vi "SeCrTs-DO Start.vi"(8 "error in":errorcluster, 9 "DO config":T1(array[cluster]), 11 "Refnum in":refnum<k21>) -> (0 "error out":errorcluster, 3 "Refnum out":refnum<k21>)   [LabVIEW 2022 SP3]
doc: "This VI is for start for Analog Output"
uses:
  RT Controls/SeCrTs-FGV Read write.ctl
  <vilib>/DAQmx/configure/timing.llb/DAQmx Timing (Sample Clock).vi
  <vilib>/DAQmx/configure/trigger.llb/DAQmx Start Trigger (Digital Edge).vi
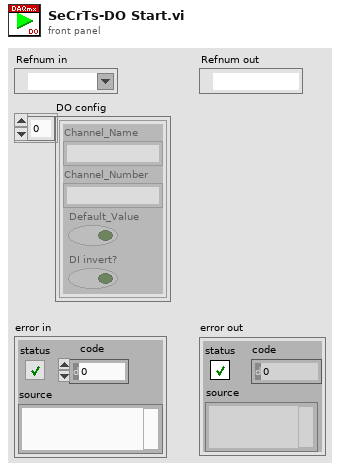
[diagram p1: front panel]
types:
  T1 = cluster{"Channel_Name":string, "Channel_Number":string, "Default_Value":bool, "DI invert?":bool}[]
  T2 = typedef "SeCrTs-FGV Read write.ctl" = enum16{"Write", "Read"}
  T3 = enum16{"Init", "Read", "Write 'All'", "Write 'n'", "Write Safe Value", "Write Start Time", "Overwrite Pattern", "Overwrite Pattern with Start", "Append Pattern", "Start Pattern Mode", "Abort Pattern Mode", "Read 1"}
  T4 = cluster{"Samples to Read":i32, "Pattern Mode?":bool, "dt(sec)":dbl, "DO Init Time (Samples)":i32, "dt per Read/Write":dbl, "Write Pointer":i32, "Pattern Size":i32, "Loop Rate (mSec)":i32, "Buffer Size (Samples)":i32, "Sampling rate":dbl, "Max DO Delay Time (samples)":dbl, "Min DO Delay Time (samples)":dbl, "Queue Size":i32, "DO Init Sample Duration (Sec)":dbl}
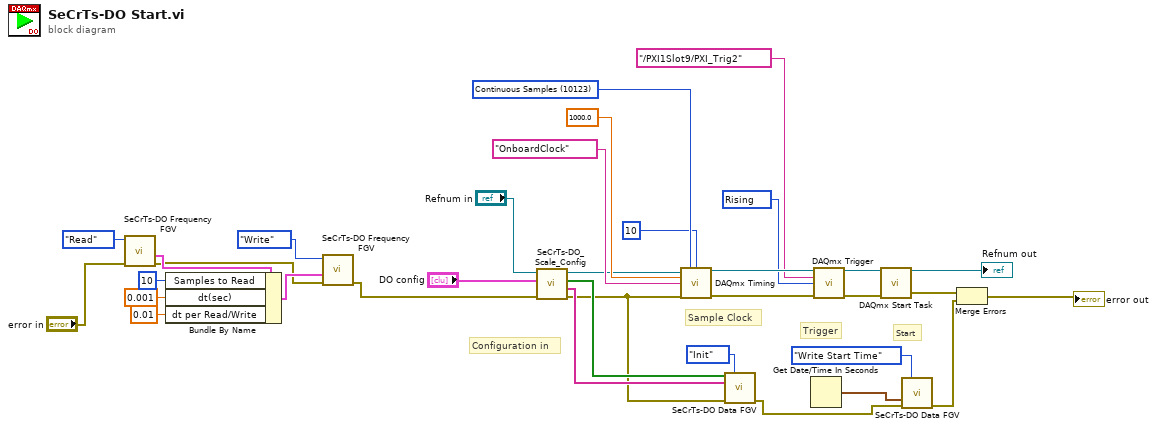
[diagram p0: block diagram]
diagram:
  w29 = 10280 items=["Rising"=10280, "Falling"=10171] ("edge")
  w26 = 10123 items=["Finite Samples"=10178, "Continuous Samples"=10123, "Hardware Timed Single Point"=12522] ("sample mode")
  # "Start"
  # "Trigger"
  # "Sample Clock"
  # "Configuration in"
  n1 = call "SeCrTs-DO Frequency  FGV.vi"("error in"="error in", "Write/Read"=SeCrTs-FGV_Read_write."Read") -> ("error in 2"=w6:errorcluster, "DO Set Frequency (R)"=w12:T4)  [unwired: 8 in]
  n2 = Bundle By Name(cluster=w12, "Samples to Read"=10, "dt(sec)"=0.001, "dt per Read/Write"=0.01) -> (w11:T4)
  n3 = call "SeCrTs-DO Frequency  FGV.vi"("error in"=w6, "DO Set Frequency (W)"=w11, "Write/Read"=SeCrTs-FGV_Read_write."Write") -> ("error in 2"=w5:errorcluster)  [unwired: 7 in, 1 out]
  n4 = call "SeCrTs-DO_Scale_Config.vi"("error in (no error)"=w5, "DO config"="DO config", "Refnum in"="Refnum in") -> ("error out"=w4:errorcluster, "Array 2"=w18:string[], "Array"=w19:bool[], "Refnum out"=w23:refnum<k21>)  [unwired: 5 in]
  n5 = call-poly <vilib>:"DAQmx Timing.vi"("task/channels in"=w23, "sample mode"=w26, "samples per channel"=10, "rate"=1000.0, "source"=tag "OnboardClock", "error in"=w4) -> ("task out"=w31:refnum<k21>, "error out"=w24:errorcluster)  [unwired: 8 in]
  n6 = call "SeCrTs-DO Data FGV.vi"("DO Values In"=w19, "Option"=T3."Init", "DO Channel Names"=w18, "error in (no error)"=w4) -> ("error out"=w15:errorcluster)  [unwired: 5 in, 6 out]
  n7 = Get Date/Time In Seconds() -> (seconds since 1Jan1904=w16:timestamp)
  n8 = call-poly <vilib>:"DAQmx Trigger.vi"("task/channels in"=w31, "source"=tag "/PXI1Slot9/PXI_Trig2", "edge"=w29, "error in"=w24) -> ("task out"=w33:refnum<k21>, "error out"=w32:errorcluster)  [unwired: 10 in]
  n9 = call <vilib>:"DAQmx Start Task.vi"("task/channels in"=w33, "error in"=w32) -> ("task out"=→"Refnum out":refnum<k21>, "error out"=w2:errorcluster)  [unwired: 12 in]
  n10 = call "SeCrTs-DO Data FGV.vi"("Option"=T3."Write Start Time", "Time Stamp In"=w16, "error in (no error)"=w15) -> ("error out"=w3:errorcluster)  [unwired: 6 in, 6 out]
  n11 = Merge Errors(w2, w3) -> (→"error out":errorcluster)
